vi "monitorXMLdoc.vi"(0 "doc":u32) -> (1 "XML-doc":string, 2 "bytes written":i32)   [LabVIEW 2019, in "Tools.lvlib" / "LibXML.lvlib"]
uses:
  LibXML.lvlib
panel:
  out "error out":errorcluster
  in  "error in":errorcluster
  out "call chain":string[](array[string])
  in  "resume":bool
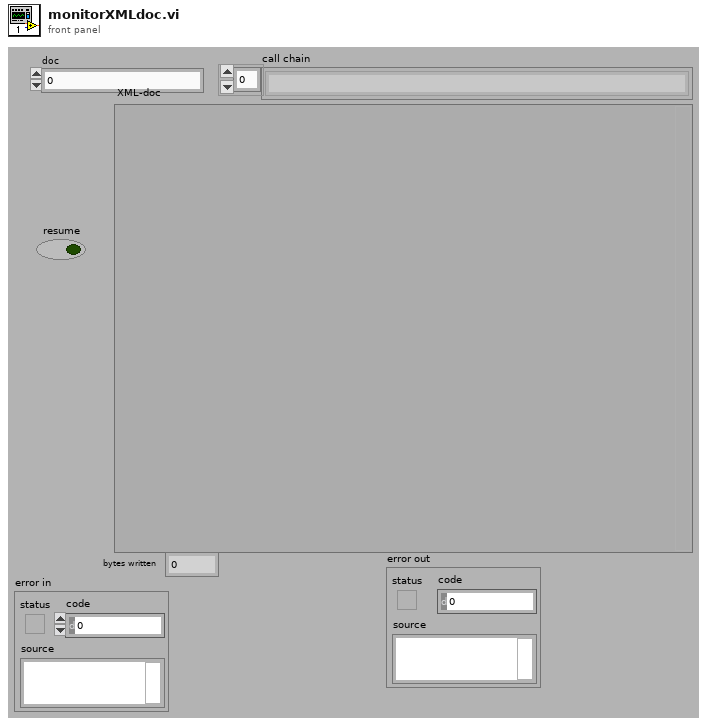
[diagram p1: front panel]
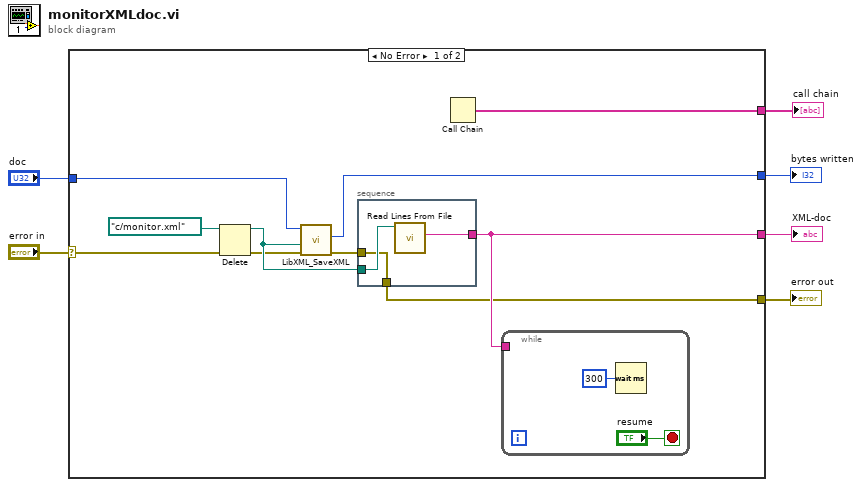
[diagram p0: block diagram]
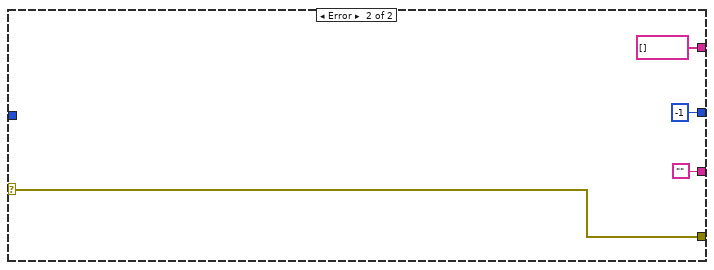
[diagram p2: hidden frame]
diagram:
  n1 = case shown="No Error" "error in" {
    selector: "error in" -> [w7 w25]
    tunnel: "doc" -> [w16 _]
    tunnel: [w13 -1 ("bytes written")] -> w5
    tunnel: [w11 string[] [] ("call chain")] -> w4
    tunnel: [w10 "" ("line string")] -> w3
    tunnel: [w8 w25] -> w2
    frame No Error {
      n2 = Delete(path (use dialog)=path "c:/monitor.xml" ("path"), error in=w7) -> (deleted path=w14:path, error out=w9:errorcluster)  [unwired: 3 in, 1 out]
      n3 = call "LibXML_SaveXML.vi"("error in"=w9, "file path (dialog if empty)"=w14, "doc"=w16) -> ("error out"=w12:errorcluster, "bytes written"=w13:i32)  [unwired: 6 in, 1 out]
      n4 = stacked-sequence {
        tunnel: w14 -> [w21]
        tunnel: [w20] -> w10
        tunnel: w12 -> [w19]
        tunnel: [w19] -> w8
        frame #0 {
          n5 = call <vilib>:"Read Lines From File.vi"("file path (dialog if empty)"=w21) -> ("line string"=w20:string)  [unwired: 5 in, 3 out]
        }
      }
      n6 = Call Chain() -> (call chain=w11:string[])
      n7 = while {
        tunnel: w10 -> [_]
        stop <- "resume" stop-if-true
        n8 = Wait (ms)(milliseconds to wait=u32 300) -> ()  [unwired: 1 out]
      }
    }
    frame Error {
    }
  }
  "XML-doc" <- w3
  "bytes written" <- w5
  "call chain" <- w4
  "error out" <- w2
